vi "Get Rectangular Coordinates.vi"(6 "method":enum16{"2 points", "4 points"}(ring), 8 "error in (no error)":errorcluster, 10 "Particle Measurements (Pixels)":dbl[](array[numeric]), 11 "Image Pixels (U8)":u8[][](array[numeric])) -> (0 "error out":errorcluster, 1 "4Side Length":dbl[](array[numeric]), 2 "4 corner Coordinates":dbl[][](array[numeric]), 3 "Distance (ft)":dbl)   [LabVIEW 2011]
uses:
  Image - 1D Search Selector.ctl
  <vilib>/Analysis/7linalg.llb/Solve Linear Equations (single right hand).vi
  <vilib>/Analysis/Matrix/Numeric/Conversions/Array To Matrix - RA2.vi
  <vilib>/Analysis/7linalg.llb/Solve Linear Eqs (General).vi
  <vilib>/Analysis/7linalg.llb/Solve Linear Eqs (Gen, single right hand).vi
  <vilib>/Analysis/NI_AALPro.lvlib
  <vilib>/Analysis/Matrix/NI_Matrix.lvlib
panel:
  in  "Tab Control":enum32{"Page 1", "Page 2"}(tab)
  out "4 corners (Local) Graph":cluster{dbl[], dbl[]}(graph)
  out "IntensityPartial":u8[][](graph)
  out "Intensity (full)":u8[][](graph)
  out "4 coners (Global) Graph 2":cluster{dbl[], dbl[]}(graph)
  out "Points on Edge Graph":cluster{dbl[], dbl[]}[](graph)
  out "Array":dbl[][](array[numeric])
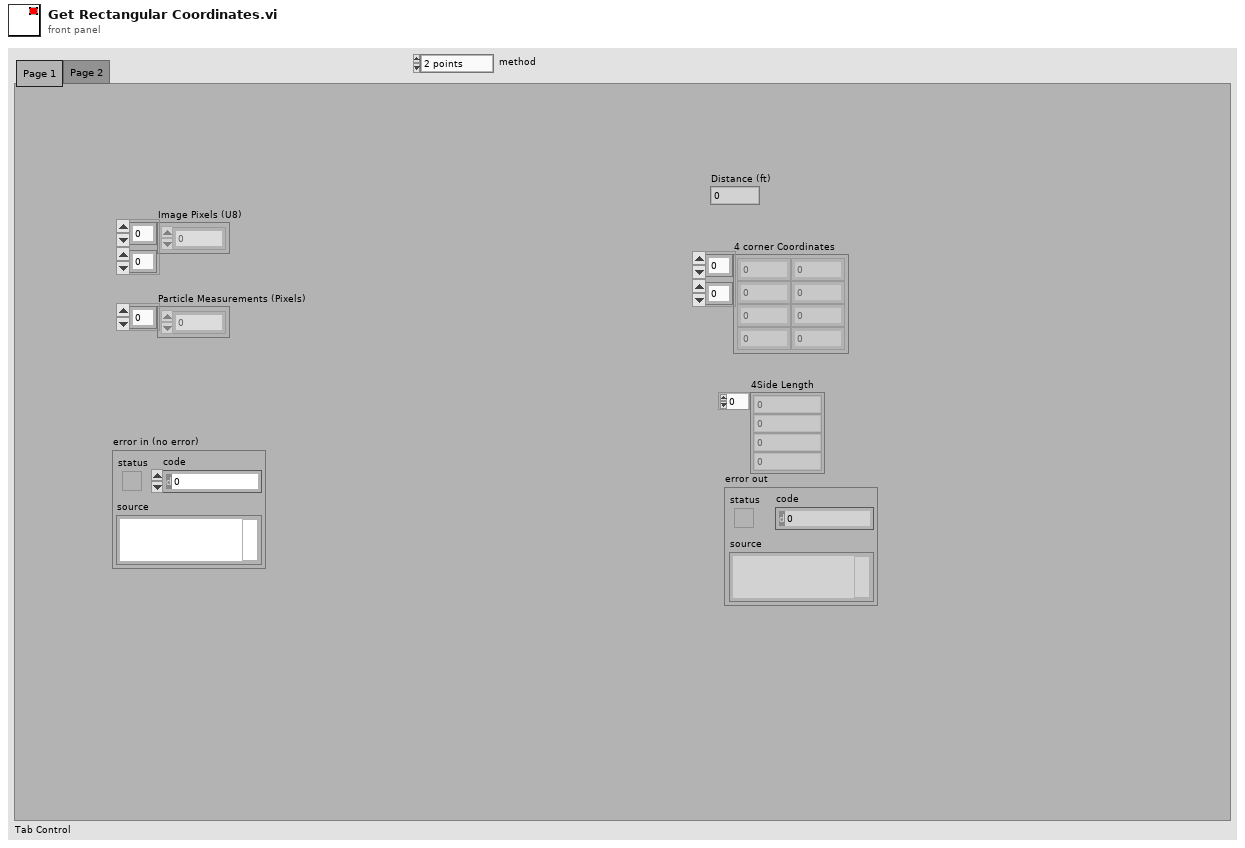
[diagram p1: front panel]
types:
  T1 = typedef "Image - 1D Search Selector.ctl" = enum16{"From Start", "From End"}
  T2 = typedef "NI_Matrix.lvlib/RealMatrix.ctl" = dbl[][]
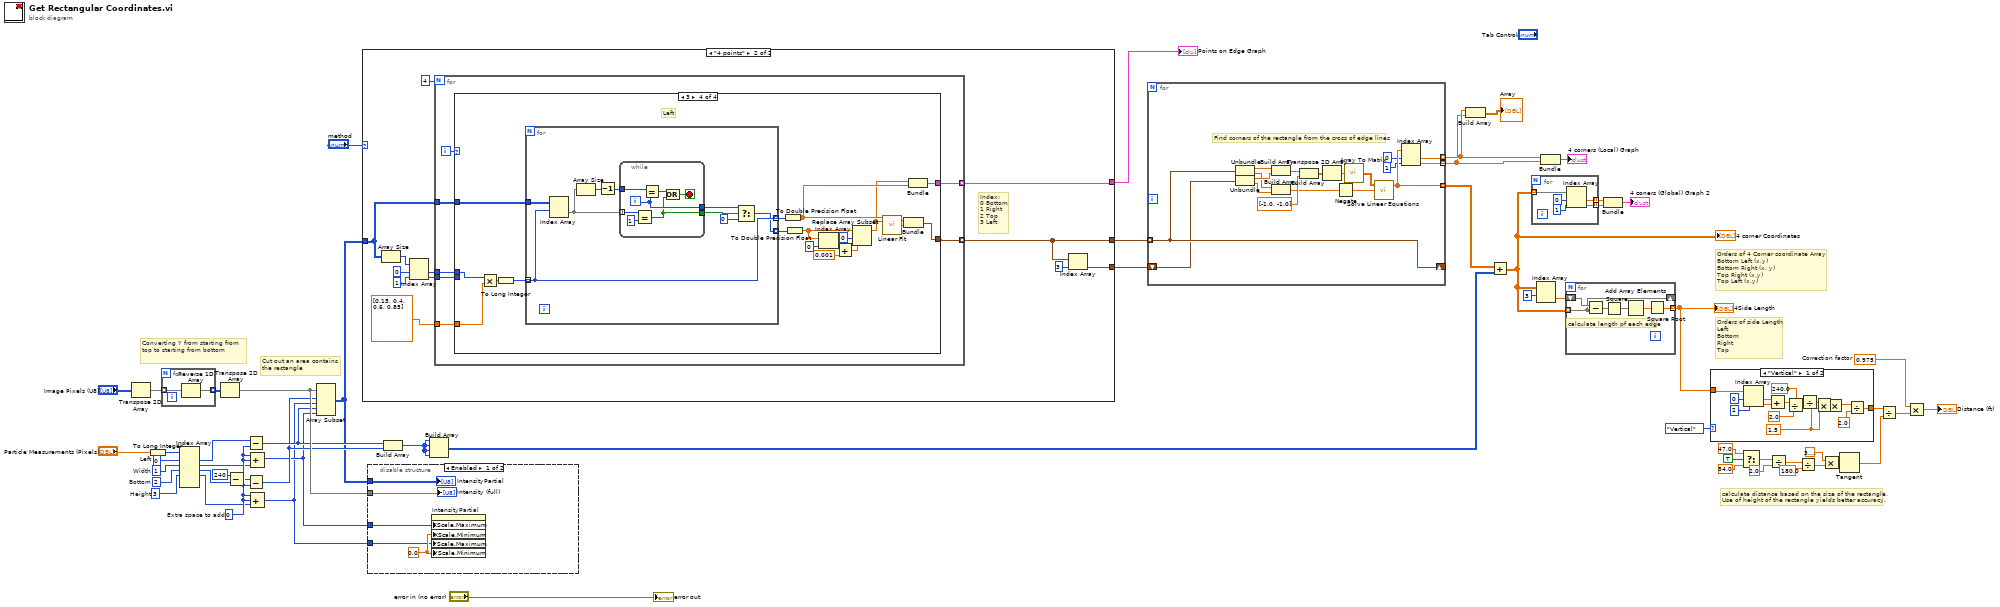
[diagram p0: block diagram]
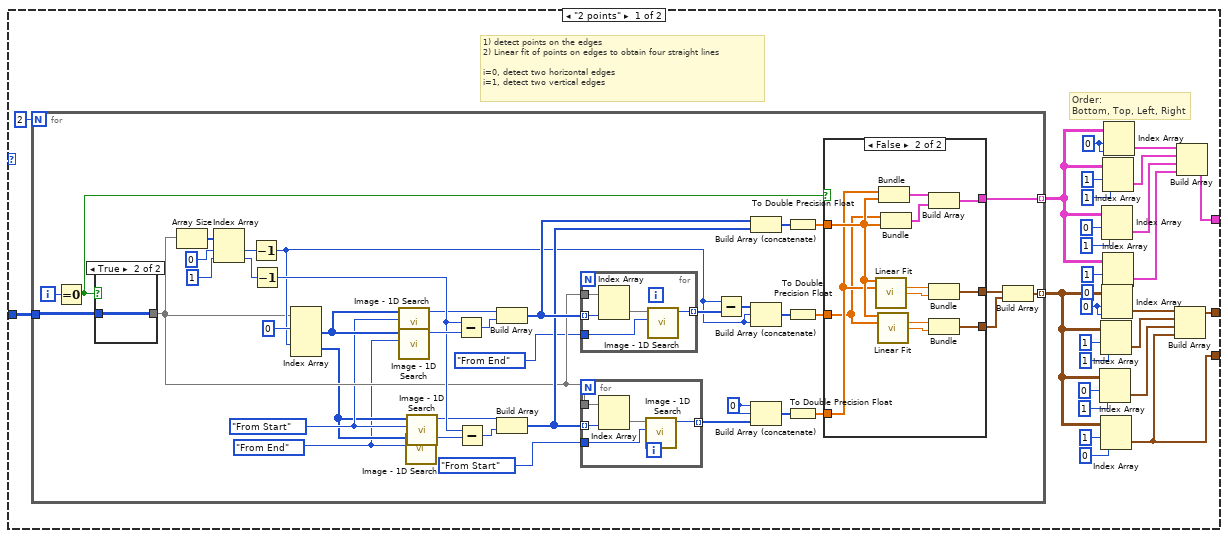
[diagram p2: hidden frame]
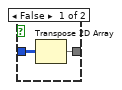
[diagram p3: hidden frame]
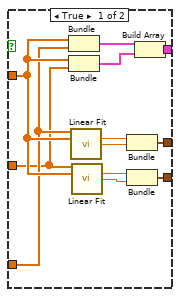
[diagram p4: hidden frame]
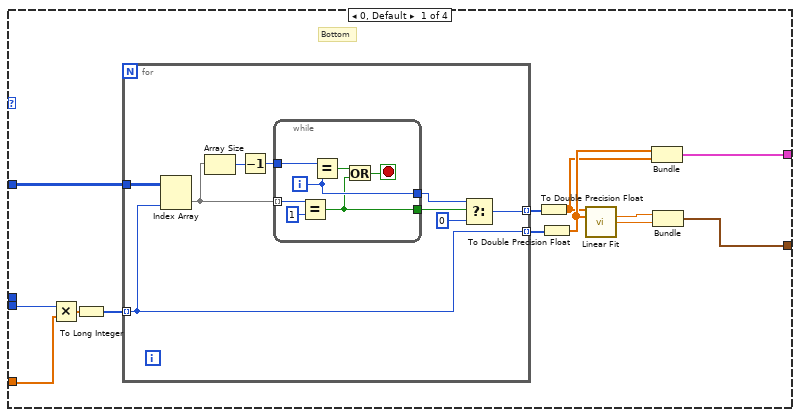
[diagram p5: hidden frame]
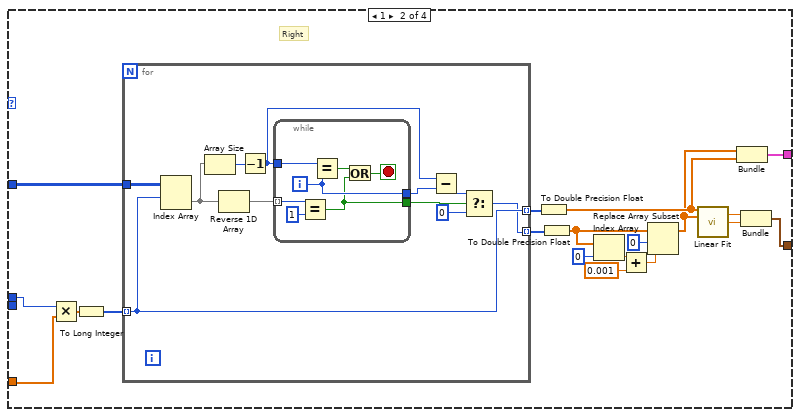
[diagram p6: hidden frame]
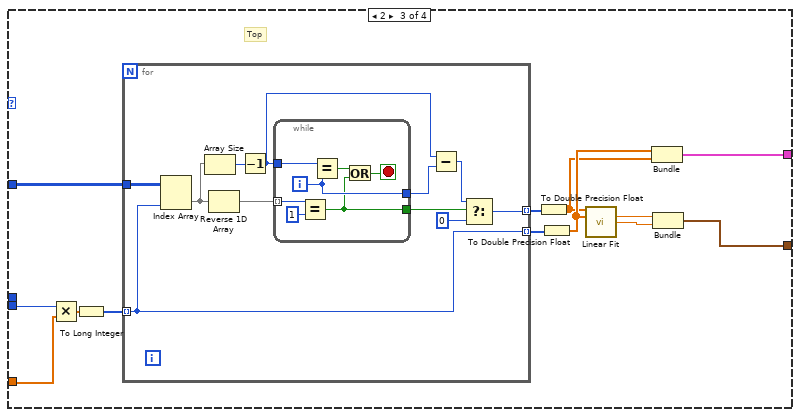
[diagram p7: hidden frame]
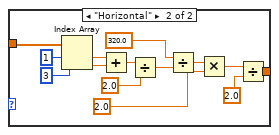
[diagram p9: hidden frame]
diagram:
  w8 = 0.975  # Correction factor
  w57 = 0  # Extra space to add
  w50 = 3  # Height
  w49 = 2  # Bottom
  w32 = 1  # Width
  w33 = 0  # Left
  # "Cut out an area contains the rectangle"
  # "Orders of side Length\nLeft\nBottom\nRight\nTop"
  # "Orders of 4 Corner coordinate Array\nBottom Left (x,y)\nBottom Right (x, y)\nTop Right (x,y)\nTop Left (x,y)"
  # "Converting Y from starting from top to starting from bottom"
  # "calculate distance based on the size of the rectangle,\nUse of height of the rectangle yields better accuracy."
  n1 = Transpose 2D Array(2D array="Image Pixels (U8)") -> (transposed array=w47:u8[][])
  n2 = To Long Integer(number="Particle Measurements (Pixels)") -> (32bit integer=w48:i32[])
  n3 = for {
    tunnel: w47 -> [w59] mode=indexing
    tunnel: [w58] -> w45 mode=indexing
    n4 = Reverse 1D Array(array=w59) -> (reversed array=w58:u8[])
  }
  n5 = Index Array(array=w48, index #1=w33, index #2=w32, index #3=w49, index #4=w50) -> (element #1=w53:i32, element #2=w54:i32, element #3=w52:i32, element #4=w56:i32)  [unwired: 2 in, 2 out]
  n6 = Transpose 2D Array(2D array=w45) -> (transposed array=w41:u8[][])
  n7 = Subtract(x=240, y=w52) -> (x-y=w55:i32)
  n8 = Subtract(x=w53, y=w57) -> (x-y=w40:i32)
  n9 = Subtract(x=w55, y=w57) -> (x-y=w34:i32)
  n10 = Compound Arithmetic op=ADD(w57, w57, w54) -> (w12:i32)
  n11 = Compound Arithmetic op=ADD(w57, w57, w56) -> (w11:i32)
  n12 = Array Subset(array=w41, index (row)=w34, length (row)=w11, index (col)=w40, length (col)=w12) -> (w5:u8[][])
  n13 = case shown="\"4 points\"" "method" {
    tunnel: [w60 w168] -> w28
    tunnel: w5 -> [w85 w172]
    tunnel: [w84 w167] -> w9
    tunnel: [w73 w166] -> w4
    frame "2 points" {
      w63 = 0 ("index (row)")
      w83 = 0 ("index (row)")
      # "Order:\nBottom, Top, Left, Right"
      # "1) detect points on the edges \n2) Linear fit of points on edges to obtain four straight lines\n\ni=0, detect two horizontal edges\ni=1, detect two vertical edges"
      n14 = for {
        N: 2 -> [_]
        tunnel: w85 -> [w102]
        tunnel: [w111] -> w76 mode=indexing
        tunnel: [w100] -> w61 mode=indexing
        i -> [w116]
        w96 = Image_-_1D_Search_Selector."From Start" ("Search Direction")
        w94 = Image_-_1D_Search_Selector."From End" ("Search Direction")
        w119 = 0
        n15 = Equal To 0?(x=w116) -> (x = 0?=w103:bool)
        n16 = case shown="True" w103 {
          tunnel: w102 -> [w129 w130]
          tunnel: [w128 w130] -> w101
          frame False {
            n17 = Transpose 2D Array(2D array=w129) -> (transposed array=w128:u8[][])
          }
          frame True {
          }
        }
        n18 = Array Size(array=w101) -> (size(s)=w125:i32[])
        n19 = Index Array(array=w125, index #1=0 ("index"), index #2=1 ("index")) -> (element #1=w124:i32, element #2=w114:i32)
        n20 = Decrement(x=w124) -> (x-1=w105:i32)
        n21 = Decrement(x=w114) -> (x-1=w118:i32)
        n22 = Index Array(array=w101, index (row) #1=0 ("index (row)"), index (row) #2=w105) -> (element #1=w99:u8[], element #2=w95:u8[])  [unwired: 2 in]
        n23 = call "Image - 1D Search.vi"("Search Direction"=w96, "Array"=w99) -> ("Index"=w98:i32)  [unwired: 9 in]
        n24 = call "Image - 1D Search.vi"("Search Direction"=w94, "Array"=w99) -> ("Index"=w126:i32)  [unwired: 9 in]
        n25 = call "Image - 1D Search.vi"("Search Direction"=w94, "Array"=w95) -> ("Index"=w93:i32)  [unwired: 9 in]
        n26 = call "Image - 1D Search.vi"("Search Direction"=w96, "Array"=w95) -> ("Index"=w97:i32)  [unwired: 9 in]
        n27 = Subtract(x=w118, y=w126) -> (x-y=w123:i32)
        n28 = Subtract(x=w118, y=w93) -> (x-y=w121:i32)
        n29 = Build Array(w98, w123) -> (w122:i32[])
        n30 = Build Array(w97, w121) -> (w120:i32[])
        n31 = for {
          tunnel: w101 -> [w164]
          tunnel: [w161] -> w106 mode=indexing
          tunnel: w122 -> [w163] mode=indexing
          tunnel: Image_-_1D_Search_Selector."From End" ("Search Direction") -> [w160]
          n32 = Index Array(array=w164, index (col)=w163) -> (element=w162:u8[])  [unwired: 1 in]
          n33 = call "Image - 1D Search.vi"("Search Direction"=w160, "Array"=w162) -> ("Index"=w161:i32)  [unwired: 9 in]
        }
        n34 = for {
          tunnel: w101 -> [w159]
          tunnel: [w156] -> w107 mode=indexing
          tunnel: w120 -> [w158] mode=indexing
          tunnel: Image_-_1D_Search_Selector."From Start" ("Search Direction") -> [w155]
          n35 = Index Array(array=w159, index (col)=w158) -> (element=w157:u8[])  [unwired: 1 in]
          n36 = call "Image - 1D Search.vi"("Search Direction"=w155, "Array"=w157) -> ("Index"=w156:i32)  [unwired: 9 in]
        }
        n37 = Subtract(x=w105, y=w106) -> (x-y=w104:i32[])
        n38 = Build Array (concatenate)(w122, w120) -> (w110:i32[])
        n39 = Build Array (concatenate)(w104, w105, w105) -> (w108:i32[])
        n40 = Build Array (concatenate)(w119, w119, w107) -> (w109:i32[])
        n41 = To Double Precision Float(number=w110) -> (double precision float=w90:dbl[])
        n42 = To Double Precision Float(number=w108) -> (double precision float=w89:dbl[])
        n43 = To Double Precision Float(number=w109) -> (double precision float=w88:dbl[])
        n44 = case shown="False" w103 {
          tunnel: w90 -> [w133 w145]
          tunnel: w88 -> [w132 w144]
          tunnel: w89 -> [w131 w143]
          tunnel: [w138 w149] -> w112
          tunnel: [w137 w152] -> w113
          tunnel: [w134 w146] -> w100
          frame True {
            n45 = Bundle(w133, w132) -> (w136:cluster{dbl[], dbl[]})  [unwired: 1 in]
            n46 = Bundle(w133, w131) -> (w135:cluster{dbl[], dbl[]})  [unwired: 1 in]
            n47 = call <vilib>:"Linear Fit.vi"("Y"=w132, "X"=w133) -> ("slope"=w142:dbl, "intercept"=w141:dbl)  [unwired: 9 in, 3 out]
            n48 = call <vilib>:"Linear Fit.vi"("Y"=w131, "X"=w133) -> ("slope"=w140:dbl, "intercept"=w139:dbl)  [unwired: 9 in, 3 out]
            n49 = Bundle("slope"=w142, "intercept"=w141) -> (w137:cluster{"slope":dbl, "intercept":dbl})  [unwired: 1 in]
            n50 = Bundle("slope"=w140, "intercept"=w139) -> (w138:cluster{"slope":dbl, "intercept":dbl})  [unwired: 1 in]
            n51 = Build Array(w136, w135) -> (w134:cluster{dbl[], dbl[]}[])
          }
          frame False {
            n52 = call <vilib>:"Linear Fit.vi"("Y"=w145, "X"=w144) -> ("slope"=w154:dbl, "intercept"=w153:dbl)  [unwired: 9 in, 3 out]
            n53 = call <vilib>:"Linear Fit.vi"("Y"=w145, "X"=w143) -> ("slope"=w151:dbl, "intercept"=w150:dbl)  [unwired: 9 in, 3 out]
            n54 = Bundle(w144, w145) -> (w148:cluster{dbl[], dbl[]})  [unwired: 1 in]
            n55 = Bundle(w143, w145) -> (w147:cluster{dbl[], dbl[]})  [unwired: 1 in]
            n56 = Build Array(w148, w147) -> (w146:cluster{dbl[], dbl[]}[])
            n57 = Bundle("slope"=w154, "intercept"=w153) -> (w152:cluster{"slope":dbl, "intercept":dbl})  [unwired: 1 in]
            n58 = Bundle("slope"=w151, "intercept"=w150) -> (w149:cluster{"slope":dbl, "intercept":dbl})  [unwired: 1 in]
          }
        }
        n59 = Build Array(w113, w112) -> (w111:cluster{"slope":dbl, "intercept":dbl}[])
      }
      n60 = Index Array(array=w76, index (row)=0, index (col)=1 ("disabled index (col)")) -> (element=w75:cluster{"slope":dbl, "intercept":dbl})
      n61 = Index Array(array=w76, index (row)=1, index (col)=1 ("disabled index (col)")) -> (element=w74:cluster{"slope":dbl, "intercept":dbl})
      n62 = Index Array(array=w76, index (row)=1, index (col)=0 ("disabled index (col)")) -> (element=w73:cluster{"slope":dbl, "intercept":dbl})
      n63 = Index Array(array=w61, index (row)=0, index (col)=1 ("disabled index (col)")) -> (element=w70:cluster{dbl[], dbl[]})
      n64 = Index Array(array=w76, index (row)=w83, index (col)=w83) -> (element=w86:cluster{"slope":dbl, "intercept":dbl})
      n65 = Index Array(array=w61, index (row)=1, index (col)=1 ("disabled index (col)")) -> (element=w71:cluster{dbl[], dbl[]})
      n66 = Index Array(array=w61, index (row)=1, index (col)=0 ("disabled index (col)")) -> (element=w72:cluster{dbl[], dbl[]})
      n67 = Index Array(array=w61, index (row)=w63, index (col)=w63) -> (element=w62:cluster{dbl[], dbl[]})
      n68 = Build Array(w86, w74, w75, w73) -> (w84:cluster{"slope":dbl, "intercept":dbl}[])
      n69 = Build Array(w62, w71, w70, w72) -> (w60:cluster{dbl[], dbl[]}[])
    }
    frame "4 points" {
      # "Index:\n0 Bottom\n1 Right\n2 Top\n3 Left"
      n70 = Array Size(array=w172) -> (size(s)=w176:i32[])
      n71 = Index Array(array=w176, index #1=0 ("index"), index #2=1 ("index")) -> (element #1=w170:i32, element #2=w171:i32)
      n72 = for {
        N: 4 -> [_]
        tunnel: w172 -> [w180]
        tunnel: w171 -> [w182]
        tunnel: w170 -> [w181]
        tunnel: dbl[] [0.15, 0.4, 0.6, 0.85] -> [w179]
        tunnel: [w178] -> w167 mode=indexing
        tunnel: [w177] -> w168 mode=indexing
        i -> [w183]
        n73 = case shown="3" w183 {
          tunnel: w182 -> [w195 _ w261 _]
          tunnel: w181 -> [_ w224 _ w288]
          tunnel: w180 -> [w192 w228 w258 w296]
          tunnel: w179 -> [w196 w231 w262 w299]
          tunnel: [w187 w225 w253 w291] -> w178
          tunnel: [w184 w223 w250 w289] -> w177
          frame 0, Default {
            # "Bottom"
            n74 = Multiply(x=w195, y=w196) -> (x*y=w194:dbl[])
            n75 = To Long Integer(number=w194) -> (32bit integer=w193:i32[])
            n76 = for {
              tunnel: w193 -> [w197] mode=indexing
              tunnel: w192 -> [w205]
              tunnel: [w198] -> w191 mode=indexing
              tunnel: [w197] -> w190 mode=indexing
              n77 = Index Array(array=w205, index (col)=w197) -> (element=w204:u8[])  [unwired: 1 in]
              n78 = Array Size(array=w204) -> (size(s)=w203:i32)
              n79 = Decrement(x=w203) -> (x-1=w202:i32)
              n80 = while {
                tunnel: w204 -> [w212] mode=indexing
                tunnel: w202 -> [w208]
                tunnel: [w207] -> w200
                tunnel: [w206] -> w201
                i -> [w207]
                stop <- w209 stop-if-true
                n81 = Equal?(x=w212, y=u8 1) -> (x = y?=w206:bool)
                n82 = Equal?(x=w208, y=w207) -> (x = y?=w210:bool)
                n83 = Or(x=w210, y=w206) -> (x .or. y?=w209:bool)
              }
              n84 = Select(t=w200, s=w201, f=0) -> (s? t:f=w198:i32)
            }
            n85 = To Double Precision Float(number=w191) -> (double precision float=w185:dbl[])
            n86 = To Double Precision Float(number=w190) -> (double precision float=w186:dbl[])
            n87 = call <vilib>:"Linear Fit.vi"("Y"=w185, "X"=w186) -> ("slope"=w189:dbl, "intercept"=w188:dbl)  [unwired: 9 in, 3 out]
            n88 = Bundle(w186, w185) -> (w184:cluster{dbl[], dbl[]})  [unwired: 1 in]
            n89 = Bundle("slope"=w189, "intercept"=w188) -> (w187:cluster{"slope":dbl, "intercept":dbl})  [unwired: 1 in]
          }
          frame 1 {
            # "Right"
            n90 = Multiply(x=w224, y=w231) -> (x*y=w230:dbl[])
            n91 = To Long Integer(number=w230) -> (32bit integer=w229:i32[])
            n92 = for {
              tunnel: w229 -> [w237] mode=indexing
              tunnel: w228 -> [w242]
              tunnel: [w237] -> w227 mode=indexing
              tunnel: [w236] -> w226 mode=indexing
              n93 = Index Array(array=w242, index (row)=w237) -> (element=w238:u8[])  [unwired: 1 in]
              n94 = Array Size(array=w238) -> (size(s)=w239:i32)
              n95 = Reverse 1D Array(array=w238) -> (reversed array=w235:u8[])
              n96 = Decrement(x=w239) -> (x-1=w233:i32)
              n97 = while {
                tunnel: w235 -> [w249] mode=indexing
                tunnel: w233 -> [w245]
                tunnel: [w244] -> w232
                tunnel: [w243] -> w241
                i -> [w244]
                stop <- w246 stop-if-true
                n98 = Equal?(x=w249, y=u8 1) -> (x = y?=w243:bool)
                n99 = Equal?(x=w245, y=w244) -> (x = y?=w247:bool)
                n100 = Or(x=w247, y=w243) -> (x .or. y?=w246:bool)
              }
              n101 = Subtract(x=w233, y=w232) -> (x-y=w234:i32)
              n102 = Select(t=w234, s=w241, f=0) -> (s? t:f=w236:i32)
            }
            n103 = To Double Precision Float(number=w227) -> (double precision float=w215:dbl[])
            n104 = To Double Precision Float(number=w226) -> (double precision float=w213:dbl[])
            n105 = Index Array(array=w213, index=0) -> (element=w219:dbl)
            n106 = Add(x=w219, y=0.001) -> (x+y=w217:dbl)
            n107 = Replace Array Subset(array=w213, new element=w217, index=0) -> (w214:dbl[])
            n108 = call <vilib>:"Linear Fit.vi"("Y"=w215, "X"=w214) -> ("slope"=w221:dbl, "intercept"=w222:dbl)  [unwired: 9 in, 3 out]
            n109 = Bundle(w214, w215) -> (w223:cluster{dbl[], dbl[]})  [unwired: 1 in]
            n110 = Bundle("slope"=w221, "intercept"=w222) -> (w225:cluster{"slope":dbl, "intercept":dbl})  [unwired: 1 in]
          }
          frame 2 {
            # "Top"
            n111 = Multiply(x=w261, y=w262) -> (x*y=w260:dbl[])
            n112 = To Long Integer(number=w260) -> (32bit integer=w259:i32[])
            n113 = for {
              tunnel: w259 -> [w268] mode=indexing
              tunnel: w258 -> [w273]
              tunnel: [w269] -> w257 mode=indexing
              tunnel: [w268] -> w256 mode=indexing
              n114 = Index Array(array=w273, index (col)=w268) -> (element=w272:u8[])  [unwired: 1 in]
              n115 = Array Size(array=w272) -> (size(s)=w266:i32)
              n116 = Reverse 1D Array(array=w272) -> (reversed array=w267:u8[])
              n117 = Decrement(x=w266) -> (x-1=w265:i32)
              n118 = while {
                tunnel: w267 -> [w280] mode=indexing
                tunnel: w265 -> [w276]
                tunnel: [w275] -> w264
                tunnel: [w274] -> w271
                i -> [w275]
                stop <- w277 stop-if-true
                n119 = Equal?(x=w280, y=u8 1) -> (x = y?=w274:bool)
                n120 = Equal?(x=w276, y=w275) -> (x = y?=w278:bool)
                n121 = Or(x=w278, y=w274) -> (x .or. y?=w277:bool)
              }
              n122 = Subtract(x=w265, y=w264) -> (x-y=w263:i32)
              n123 = Select(t=w263, s=w271, f=0) -> (s? t:f=w269:i32)
            }
            n124 = To Double Precision Float(number=w257) -> (double precision float=w251:dbl[])
            n125 = To Double Precision Float(number=w256) -> (double precision float=w252:dbl[])
            n126 = call <vilib>:"Linear Fit.vi"("Y"=w251, "X"=w252) -> ("slope"=w255:dbl, "intercept"=w254:dbl)  [unwired: 9 in, 3 out]
            n127 = Bundle(w252, w251) -> (w250:cluster{dbl[], dbl[]})  [unwired: 1 in]
            n128 = Bundle("slope"=w255, "intercept"=w254) -> (w253:cluster{"slope":dbl, "intercept":dbl})  [unwired: 1 in]
          }
          frame 3 {
            # "Left"
            n129 = Multiply(x=w288, y=w299) -> (x*y=w298:dbl[])
            n130 = To Long Integer(number=w298) -> (32bit integer=w297:i32[])
            n131 = for {
              tunnel: w297 -> [w301] mode=indexing
              tunnel: w296 -> [w308]
              tunnel: [w301] -> w295 mode=indexing
              tunnel: [w300] -> w294 mode=indexing
              n132 = Index Array(array=w308, index (row)=w301) -> (element=w302:u8[])  [unwired: 1 in]
              n133 = Array Size(array=w302) -> (size(s)=w305:i32)
              n134 = Decrement(x=w305) -> (x-1=w304:i32)
              n135 = while {
                tunnel: w302 -> [w315] mode=indexing
                tunnel: w304 -> [w311]
                tunnel: [w310] -> w303
                tunnel: [w309] -> w307
                i -> [w310]
                stop <- w312 stop-if-true
                n136 = Equal?(x=w315, y=u8 1) -> (x = y?=w309:bool)
                n137 = Equal?(x=w311, y=w310) -> (x = y?=w313:bool)
                n138 = Or(x=w313, y=w309) -> (x .or. y?=w312:bool)
              }
              n139 = Select(t=w303, s=w307, f=0) -> (s? t:f=w300:i32)
            }
            n140 = To Double Precision Float(number=w295) -> (double precision float=w290:dbl[])
            n141 = To Double Precision Float(number=w294) -> (double precision float=w283:dbl[])
            n142 = Index Array(array=w283, index=0) -> (element=w286:dbl)
            n143 = Add(x=w286, y=0.001) -> (x+y=w285:dbl)
            n144 = Replace Array Subset(array=w283, new element=w285, index=0) -> (w282:dbl[])
            n145 = call <vilib>:"Linear Fit.vi"("Y"=w290, "X"=w282) -> ("slope"=w293:dbl, "intercept"=w292:dbl)  [unwired: 9 in, 3 out]
            n146 = Bundle("slope"=w293, "intercept"=w292) -> (w291:cluster{"slope":dbl, "intercept":dbl})  [unwired: 1 in]
            n147 = Bundle(w282, w290) -> (w289:cluster{dbl[], dbl[]})  [unwired: 1 in]
          }
        }
      }
      n148 = Index Array(array=w167, index=3) -> (element=w166:cluster{"slope":dbl, "intercept":dbl})
    }
  }
  "Points on Edge Graph" <- w28
  n149 = disable-structure shown="Enabled" {
    disable-tunnel: w5 -> [w320 _]
    disable-tunnel: w41 -> [w319 _]
    disable-tunnel: w12 -> [w316 _]
    disable-tunnel: w11 -> [w317 _]
    frame Enabled {
      w318 = 0.0 ("X Scale.Range:Minimum")
      n150 = property on="IntensityPartial" class="IntGraph (strict)"("XScale.Maximum"=w316, "XScale.Minimum"=w318, "YScale.Maximum"=w317, "YScale.Minimum"=w318) -> ()  [unwired: 2 in, 2 out]
      "IntensityPartial" <- w320
      "Intensity (full)" <- w319
    }
    frame Disabled {
    }
  }
  n151 = Build Array(w40, w34) -> (w27:i32[])
  n152 = Build Array(w27, w27, w27, w27) -> (w38:i32[][])
  n153 = for {
    tunnel: w9 -> [w322] mode=indexing
    tunnel: [w327] -> w39 mode=indexing
    tunnel: [w324] -> w44 mode=indexing
    tunnel: [w323] -> w1 mode=indexing
    shift-right: [w322] -> _
    shift-left: w4 -> [w321]
    # "Find corners of the rectangle from the cross of edge lines"
    n154 = Unbundle(w322) -> ("slope"=w338:dbl, "intercept"=w336:dbl)
    n155 = Unbundle(w321) -> ("slope"=w337:dbl, "intercept"=w335:dbl)
    n156 = Build Array(w338, w337) -> (w334:dbl[])
    n157 = Build Array(w336, w335) -> (w331:dbl[])
    n158 = Build Array(w334, dbl[] [-1.0, -1.0]) -> (w332:dbl[][])
    n159 = Transpose 2D Array(2D array=w332) -> (transposed array=w329:dbl[][])
    n160 = Negate(x=w331) -> (-x=w328:dbl[])
    n161 = call-poly <vilib>:"Array To Matrix.vi"("Real 2D Array"=w329) -> ("Real Matrix"=w330:T2)
    n162 = call-poly <vilib>:"Solve Linear Equations.vi"("Known Vector"=w328, "Input Matrix"=w330) -> ("Solution Vector"=w327:dbl[])  [unwired: 1 in, 1 out]
    n163 = Index Array(array=w327, index #1=0 ("index"), index #2=1 ("index")) -> (element #1=w324:dbl, element #2=w323:dbl)
  }
  n164 = Build Array(w44, w1) -> (→"Array":dbl[][])
  n165 = Add(x=w39, y=w38) -> (x+y=w31:dbl[][])
  "4 corner Coordinates" <- w31
  n166 = for {
    tunnel: w31 -> [w341] mode=indexing
    tunnel: [w340] -> w36 mode=indexing
    tunnel: [w339] -> w35 mode=indexing
    n167 = Index Array(array=w341, index #1=0 ("index"), index #2=1 ("index")) -> (element #1=w340:dbl, element #2=w339:dbl)
  }
  n168 = Index Array(array=w31, index (row)=3) -> (element=w29:dbl[])  [unwired: 1 in]
  n169 = Bundle(w44, w1) -> (→"4 corners (Local) Graph":cluster{dbl[], dbl[]})  [unwired: 1 in]
  n170 = for {
    tunnel: w31 -> [w344] mode=indexing
    shift-right: [w344] -> _
    shift-left: w29 -> [w345]
    tunnel: [w346] -> w13 mode=indexing
    # "calculate length pf each edge"
    n171 = Subtract(x=w345, y=w344) -> (x-y=w349:dbl[])
    n172 = Square(x=w349) -> (x^2=w348:dbl[])
    n173 = Add Array Elements(numeric array=w348) -> (sum=w347:dbl)
    n174 = Square Root(x=w347) -> (sqrt(x)=w346:dbl)
  }
  "4Side Length" <- w13
  n175 = Bundle(w36, w35) -> (→"4 coners (Global) Graph 2":cluster{dbl[], dbl[]})  [unwired: 1 in]
  n176 = case shown="\"Vertical\"" enum16{"Horizontal", "Vertical"}."Vertical" ("Enum") {
    tunnel: w13 -> [w364 w378]
    tunnel: [w352 w365] -> w19
    frame "Vertical" {
      w350 = 1.5
      n177 = Index Array(array=w364, index #1=0 ("index"), index #2=2 ("index")) -> (element #1=w360:dbl, element #2=w361:dbl)
      n178 = Add(x=w360, y=w361) -> (x+y=w359:dbl)
      n179 = Divide(x=w359, y=2.0) -> (x/y=w356:dbl)
      n180 = Divide(x=240.0, y=w356) -> (x/y=w355:dbl)
      n181 = Multiply(x=w355, y=w350) -> (x*y=w354:dbl)
      n182 = Multiply(x=w354, y=w350) -> (x*y=w351:dbl)
      n183 = Divide(x=w351, y=2.0) -> (x/y=w352:dbl)
    }
    frame "Horizontal" {
      n184 = Index Array(array=w378, index #1=1 ("index"), index #2=3 ("index")) -> (element #1=w374:dbl, element #2=w375:dbl)
      n185 = Add(x=w374, y=w375) -> (x+y=w373:dbl)
      n186 = Divide(x=w373, y=2.0) -> (x/y=w370:dbl)
      n187 = Divide(x=320.0, y=w370) -> (x/y=w369:dbl)
      n188 = Multiply(x=w369, y=2.0) -> (x*y=w367:dbl)
      n189 = Divide(x=w367, y=2.0) -> (x/y=w365:dbl)
    }
  }
  n190 = Select(t=47.0, s=TRUE, f=54.0) -> (s? t:f=w16:dbl)
  n191 = Divide(x=w16, y=2.0) -> (x/y=w17:dbl)
  n192 = Divide(x=w17, y=180.0) -> (x/y=w22:dbl)
  n193 = Multiply(x=3.141592653589793, y=w22) -> (x*y=w20:dbl)
  n194 = Tangent(1:w20) -> (0:w18:dbl)
  n195 = Divide(x=w19, y=w18) -> (x/y=w7:dbl)
  n196 = Multiply(x=w8, y=w7) -> (x*y=→"Distance (ft)":dbl)
  "error out" <- "error in (no error)"
